vi "MRB_auto_ctrl_with_magnet_pressure.vi"(4 "ref_reinit":refnum<vi>, 6 "ref_sp_ch1":refnum<vi>, 7 "array_value_in":dbl[](array[numeric]), 9 "P_set":dbl=0.5 caption="Set Point" format="%#_13g", 10 "enable_auto_ctrl":bool caption="Auto Control") -> (0 "F_new":dbl format="%.3f", 1 "auto_ctrl_status":u32(colorbox) caption="Status", 2 "P_psi":dbl=1.1 format="%.2f", 3 "P_Torr":dbl=1.1 format="%.1f", 5 "array_value_out":dbl[](array[numeric]))   [LabVIEW 2019]
doc: "This example demonstrates how to simulate a general PID controller."
uses:
  <vilib>/Analysis/baseanly.llb/Mean (DBL).vi
  MaxiGauge/MaxiGauge_Global.vi
  <vilib>/addons/control/pid/pid.llb/PID (DBL).vi
  <vilib>/addons/control/pid/NI_PID_pid.lvlib
  <vilib>/Analysis/NI_AALBase.lvlib
panel:
  in  "sp_step":dbl=1.0 format="%#_13g"
  in  "sp_nominal":dbl=5.0
  in  "sp_max":dbl=20.0
  in  "sp_min":dbl
  in  "n_avg":u8=10
  out "MV":dbl format="%.1f"
  in  "P_max":dbl=1.4 format="%.1f"
  in  "P_min":dbl=-0.4 format="%.1f"
  out "PID Range":cluster{"High":dbl, "Low":dbl}={"High"=20.0, "Low"=-20.0} {"Low" format="%.1f"; "High" format="%.1f"}
  in  "PID gains":T1={"proportional gain (Kc)"=-10.0, "integral time (Ti, min)"=0.2, "derivative time (Td, min)"=0.1} {"derivative time (Td, min)" format="%.4f"; "integral time (Ti, min)" format="%.4f"; "proportional gain (Kc)" format="%.3f"}
  # "psi"
  # "psi"
  # "K_c = dO/dP = -1.0/0.1 = -10.0\nT_i = 1.0 (was 0.2)\nT_d = 0.2 (was 0.1)"
  # "L/m"
  # "L/m"
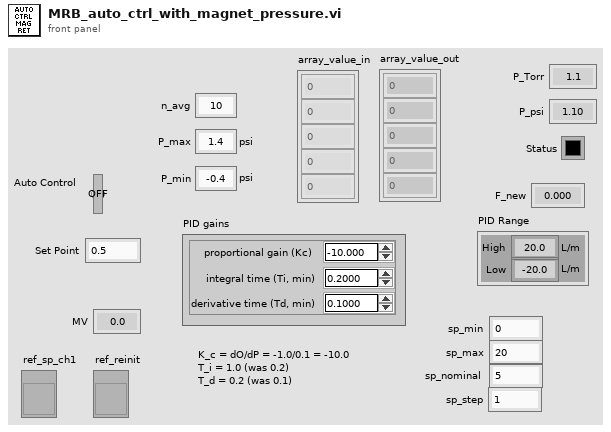
[diagram p1: front panel]
types:
  T1 = cluster{"proportional gain (Kc)":dbl, "integral time (Ti, min)":dbl, "derivative time (Td, min)":dbl}
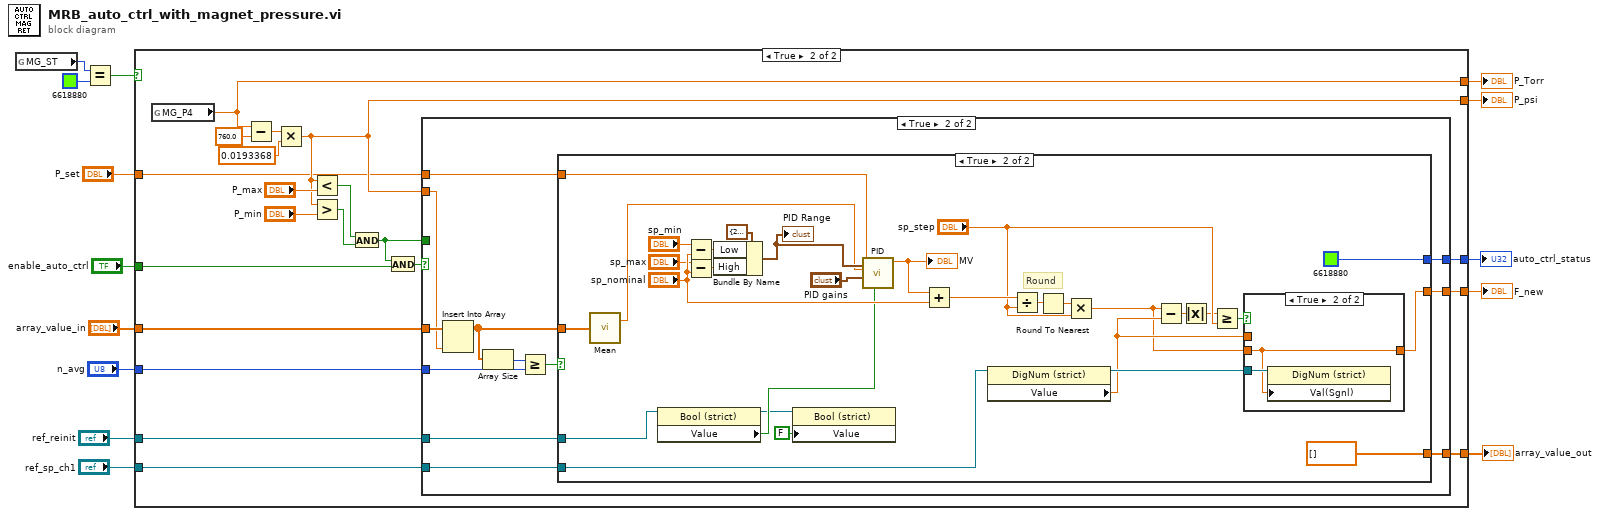
[diagram p0: block diagram]
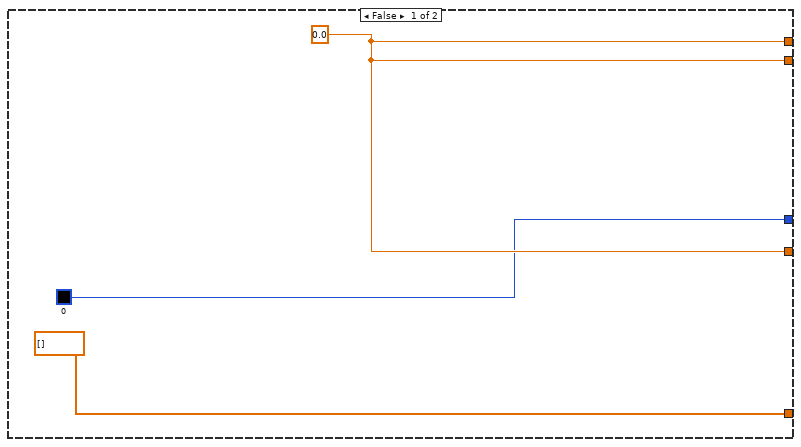
[diagram p2: hidden frame]
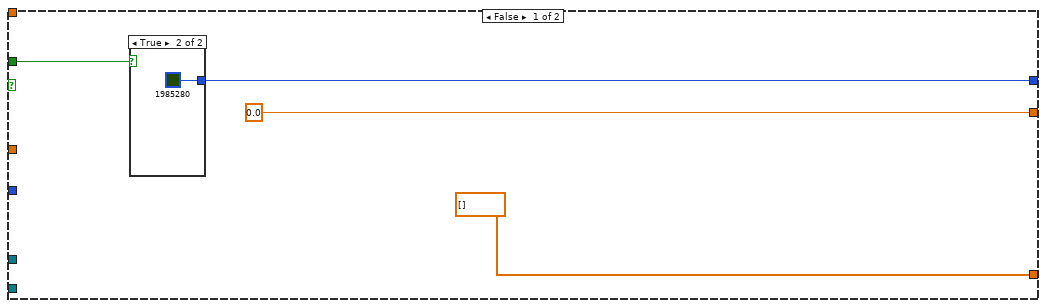
[diagram p3: hidden frame]
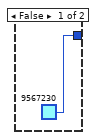
[diagram p4: hidden frame]
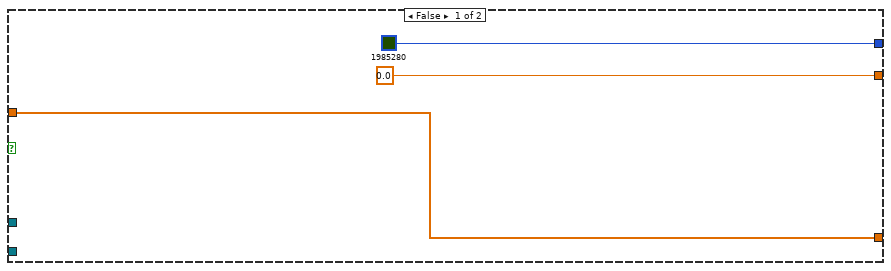
[diagram p5: hidden frame]
diagram:
  n1 = global read "MaxiGauge_Global.vi" "MG_ST"() -> (w3:u32)
  n2 = Equal?(x=w3, y=u32 6618880 ("MG_ST")) -> (x = y?=w1:bool)
  n3 = case shown="True" w1 {
    tunnel: [w17 w37] -> w14
    tunnel: [u32 0 ("alarm_status") w36] -> w13
    tunnel: "P_set" -> [_ w22]
    tunnel: "enable_auto_ctrl" -> [_ w27]
    tunnel: [w17 w18] -> w10
    tunnel: [w17 w30] -> w9
    tunnel: "ref_sp_ch1" -> [_ w29]
    tunnel: "ref_reinit" -> [_ w23]
    tunnel: "array_value_in" -> [_ w21]
    tunnel: "n_avg" -> [_ w20]
    tunnel: [dbl[] [] ("f") w19] -> w4
    frame False {
      w17 = 0.0 ("Value")
    }
    frame True {
      n4 = global read "MaxiGauge_Global.vi" "MG_P4"() -> (w18:dbl)
      n5 = Subtract(x=w18, y=760.0) -> (x-y=w34:dbl)
      n6 = Multiply(x=w34, y=0.0193368) -> (x*y=w30:dbl)
      n7 = Less?(x=w30, y="P_max") -> (x < y?=w25:bool)
      n8 = Greater?(x=w30, y="P_min") -> (0:w26:bool)
      n9 = And(x=w25, y=w26) -> (x .and. y?=w24:bool)
      n10 = And(x=w24, y=w27) -> (x .and. y?=w28:bool)
      n11 = case shown="True" w28 {
        tunnel: [0.0 ("F_O_new") w53] -> w37
        tunnel: [w39 w55] -> w36
        tunnel: w22 -> [_ w52]
        tunnel: w30 -> [_ w49]
        tunnel: w29 -> [_ w54]
        tunnel: w24 -> [w40 _]
        tunnel: w23 -> [_ w51]
        tunnel: w21 -> [_ w50]
        tunnel: w20 -> [_ w47]
        tunnel: [dbl[] [] ("f") w44] -> w19
        frame False {
          n12 = case shown="True" w40 {
            tunnel: [u32 9567230 ("alarm_status") u32 1985280 ("alarm_status")] -> w39
            frame False {
            }
            frame True {
            }
          }
        }
        frame True {
          n13 = Insert Into Array(array=w50, new element=w49) -> (w45:dbl[])  [unwired: 1 in]
          n14 = Array Size(array=w45) -> (size(s)=w48:i32)
          n15 = Greater Or Equal?(x=w48, y=w47) -> (x >= y?=w46:bool)
          n16 = case shown="True" w46 {
            tunnel: [u32 1985280 ("alarm_status") u32 6618880 ("alarm_status")] -> w55
            tunnel: w54 -> [_ w87]
            tunnel: [0.0 ("F_new") w86] -> w53
            tunnel: w52 -> [_ w84]
            tunnel: w51 -> [_ w82]
            tunnel: w45 -> [w56 w71]
            tunnel: [w56 dbl[] [] ("f")] -> w44
            frame False {
            }
            frame True {
              # "Round"
              n17 = call-poly <vilib>:"Mean.vi"("X"=w71) -> ("mean"=w70:dbl)  [unwired: 1 out]
              n18 = property class="Bool (strict)"(reference=w82) -> (reference out=w80:refnum<vi>, "Value"=w81:bool)  [unwired: 1 in, 1 out]
              n19 = Subtract(x="sp_min", y="sp_nominal") -> (x-y=w76:dbl)
              n20 = Subtract(x="sp_max", y="sp_nominal") -> (x-y=w77:dbl)
              n21 = Bundle By Name(cluster=cluster{"High":dbl, "Low":dbl} {"High"=20.0, "Low"=-20.0} ("PID Range"), "Low"=w76, "High"=w77) -> (w72:cluster{"High":dbl, "Low":dbl})
              "PID Range" <- w72
              n22 = property class="Bool (strict)"(reference=w80, "Value"=FALSE) -> ()  [unwired: 1 in, 2 out]
              n23 = call-poly <vilib>:"PID.vi"("reinitialize? (F)"=w81, "output range"=w72, "PID gains"="PID gains", "process variable"=w70, "setpoint"=w84) -> ("output"=w83:dbl)  [unwired: 5 in, 1 out]
              "MV" <- w83
              n24 = Add(x=w83, y="sp_nominal") -> (x+y=w66:dbl)
              n25 = property class="DigNum (strict)"(reference=w87) -> ("Value"=w68:dbl)  [unwired: 1 in, 2 out]
              n26 = Divide(x=w66, y="sp_step") -> (x/y=w63:dbl)
              n27 = Round To Nearest(number=w63) -> (nearest integer value=w64:dbl)
              n28 = Multiply(x=w64, y="sp_step") -> (x*y=w67:dbl)
              n29 = Subtract(x=w67, y=w68) -> (x-y=w60:dbl)
              n30 = Absolute Value(x=w60) -> (abs(x)=w61:dbl)
              n31 = Greater Or Equal?(x=w61, y="sp_step") -> (x >= y?=w62:bool)
              n32 = case shown="True" w62 {
                tunnel: w87 -> [_ w90]
                tunnel: w67 -> [_ w89]
                tunnel: [w88 w89] -> w86
                tunnel: w68 -> [w88 _]
                frame False {
                }
                frame True {
                  n33 = property class="DigNum (strict)"(reference=w90, "Val(Sgnl)"=w89) -> ()  [unwired: 1 in, 2 out]
                }
              }
            }
          }
        }
      }
    }
  }
  "F_new" <- w14
  "auto_ctrl_status" <- w13
  "P_Torr" <- w10
  "P_psi" <- w9
  "array_value_out" <- w4
